vi "RemoveGLFInstance.vi"(8 "error in (no error)":errorcluster, 10 "GLF Instance":refnum<class "IAmGLF.lvclass">, 11 "Engine in":refnum<class "Engine.lvclass">) -> (0 "error out":errorcluster, 3 "Engine out":refnum<class "Engine.lvclass">)   [LabVIEW 2024, in "GLF.lvlib" / "Engine.lvclass"]
uses:
  Engine.lvclass
  IAmGLF/IAmGLF.lvclass
  Engine.lvclass/Engine.ctl
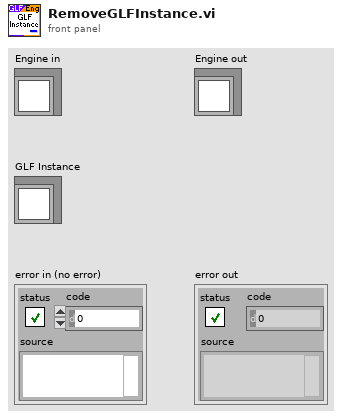
[diagram p1: front panel]
types:
  T1 = typedef "GLF.lvlib/Engine.lvclass/DVR--cluster.ctl" = cluster{"CMD Queue":T2, "Config":T3, "Ctxt":T5, "Metrics":T6, "GLF Instances":set{refnum<class "IAmGLF.lvclass">}, "Window Instances":map{i64, refnum<class "Window.lvclass">}}
  T2 = typedef "GLF.lvlib/Engine.lvclass/Command--queue.ctl" = refnum<queue>
  T3 = typedef "GLF.lvlib/Engine.lvclass/Config--cluster.ctl" = cluster{"Quit On Last Window Closed":bool, "VSync":T4, "FPS Target":dbl}
  T4 = typedef "GLF.lvlib/Engine.lvclass/VSync--enum.ctl" = enum16{"Disabled", "Enabled", "Adaptative"}
  T5 = typedef "GLF.lvlib/Engine.lvclass/Context--cluster.ctl" = cluster{"Ticks Begin":u64, "VSync Enabled":bool}
  T6 = typedef "GLF.lvlib/Engine.lvclass/Metrics--cluster.ctl" = cluster{"Uptime [ms]":u64, "Loop Time [ms]":u64}
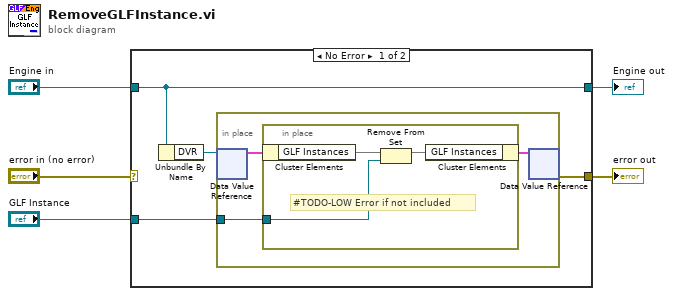
[diagram p0: block diagram]
diagram:
  n1 = case shown="No Error" "error in (no error)" {
    selector: "error in (no error)" -> [_ w17]
    tunnel: [w7 w17] -> w4
    tunnel: [w9 w16] -> w2
    tunnel: "Engine in" -> [w9 w16]
    tunnel: "GLF Instance" -> [w6 _]
    frame No Error {
      n2 = Unbundle By Name(w9) -> ("DVR"=w8:refnum<data-value>)
      n3 = in-place {
        in-place-border: w6 -> [w10]
        n4 = in-place-dvr #1(w8) -> (w12:T1)  [unwired: 1 out]
        n5 = in-place {
          in-place-border: w10 -> [w13]
          # "#TODO-LOW Error if not included"
          n6 = in-place-cluster #2(w12) -> ("GLF Instances"=w15:set{refnum<class "IAmGLF.lvclass">})
          n7 = Remove From Set(10:w13, 11:w15) -> (3:w14:set{refnum<class "IAmGLF.lvclass">})  [unwired: 1 out]
          n8 = in-place-cluster #2("GLF Instances"=w14) -> (w11:T1)
        }
        n9 = in-place-dvr #1(w11) -> (w7:errorcluster)  [unwired: 1 out]
      }
    }
    frame Error {
    }
  }
  "error out" <- w4
  "Engine out" <- w2
